vi "Plot_Many_Channels.vi"() -> (5 "Plug in titles":string[](array[string]), 7 "Plug in values":string[](array[string]))   [LabVIEW 2021]
uses:
  07834b75-344c-4d4c-a66e-07bf327eec95.vi
  Globals/Meas_global.vi
  <vilib>/Analysis/NI_AALBase.lvlib
panel:
  in  "Display:":enum16{"Show All", "My Choice", "Hide All"}(ring)
  in  "Plot:":enum16{"Eng. Units", "Voltages"}(ring)
  out "XY Graph":cluster{"Time (s)":dbl[], "Voltage":dbl[]}[](graph)
  # "Channel"
  # "Value"
  # "Voltage"
  # "StdDev(V)"
  # "Name"
  # "Symbol"
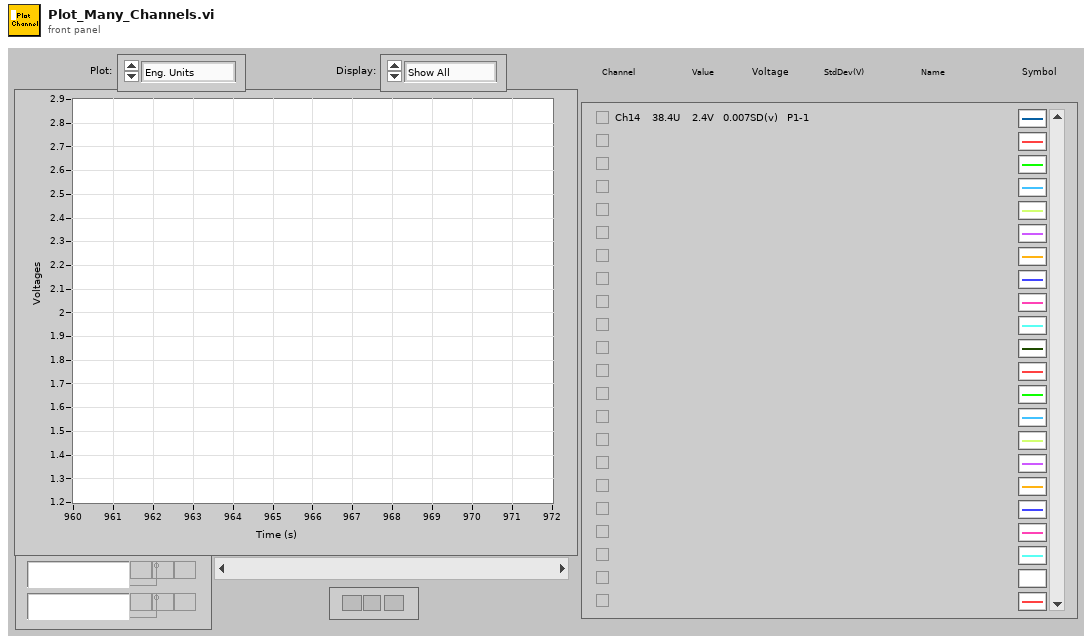
[diagram p1: front panel]
types:
  T1 = typedef "Analysis_info_cluster.ctl" = cluster{"Colour":u32, "Inst type":T2, "Inst name":string, "Symbol":string, "Code name":string, "Extra Info":string, "Inst Array":T3, "Extra Titles":string[], "Extra Values":string[], "U":dbl, "u^2":dbl, "u^3":dbl, "u^4":dbl, "Skew_u":dbl, "Kurt_u":dbl, "Sd Error in Mean":dbl, "% u'/U":dbl, "X":dbl, "Y":dbl, "Z":dbl, "Timescale integral Estimate":dbl, "Sd Error in Variance":dbl, "Calib File":path, "Calib Constants":dbl[], "Output Position":bool, "Stats":enum16{"None", "Basic", "Full"}, "Av Sampling Rate":dbl, "Av No of Samples":dbl, "Total Meas Time (s)":dbl, "ADAM Ch Name":string, "Max value":dbl, "Min value":dbl, "Req Sample Rate Hz":dbl, "Sync Delay Time (s)":dbl, "Ch No":i16, "Device":string, "Use Latest Calib":bool, "Port":string, "Metadata Ch Names":string[], "Metadata Ch Values":string[], "Label":string}
  T2 = typedef "Inst_type.ctl" = enum16{"Raw voltage", "Raw with zero offsetting", "Propeller anemometer", "Pressure Transducer", "Pitot-static tube", "Hot wire", "Cross wire 1", "Cross wire 2", "Generic Linear", "Generic Polynomial", "Generic BackPoly", "Fast FID", "Thermocouple", "Cold wire", "Pulsed Wire", "LDA Vel", "LDA Tran time", "LDA Arr time", "Microphone"}
  T3 = typedef "Instrument_Array.ctl" = enum16{"PWA", "LDA", "Analogue"}
  T4 = typedef "Time_Trace_Cluster.ctl" = cluster{"Weighting":dbl[], "Voltage":dbl[], "Eng Values":dbl[]}
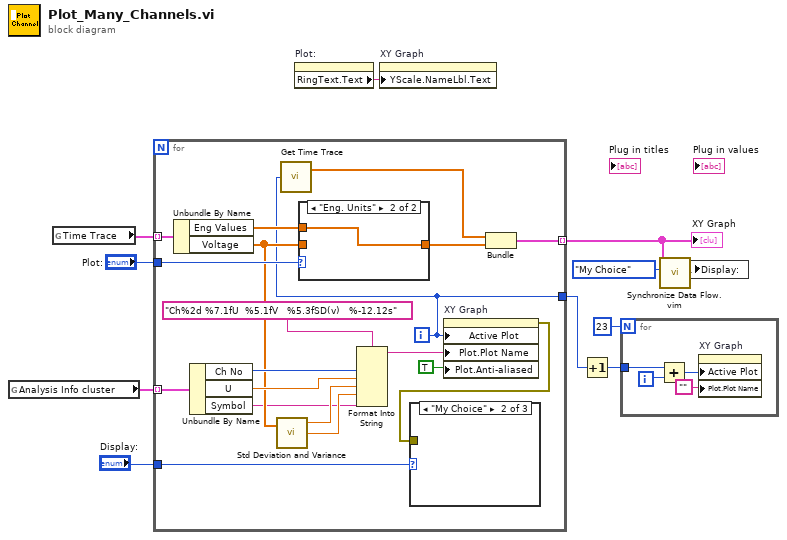
[diagram p0: block diagram]
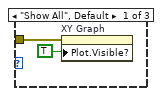
[diagram p2: hidden frame]
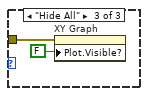
[diagram p3: hidden frame]
diagram:
  n1 = global read "Meas_global.vi" "Analysis Info cluster"() -> (w11:T1[])
  n2 = global read "Meas_global.vi" "Time Trace"() -> (w8:T4[])
  n3 = for {
    tunnel: [w30] -> w5 mode=indexing
    tunnel: w11 -> [w29] mode=indexing
    tunnel: "Plot:" -> [w28]
    tunnel: "Display:" -> [w15]
    tunnel: w8 -> [w14] mode=indexing
    tunnel: [w13] -> w3
    i -> [w13]
    n4 = Unbundle By Name(w14) -> ("Eng Values"=w21:dbl[], "Voltage"=w20:dbl[])
    n5 = Unbundle By Name(w29) -> ("Ch No"=w26:i16, "U"=w25:dbl, "Symbol"=w17:string)
    n6 = call <vilib>:"Std Deviation and Variance.vi"("X"=w20) -> ("mean"=w19:dbl, "standard deviation"=w18:dbl)  [unwired: 1 in, 1 out]
    n7 = call "Get Time Trace.vi"("Channel Index"=w13) -> ("Time (s)"=w12:dbl[])  [unwired: 1 out]
    n8 = case shown="\"Eng. Units\"" w28 {
      tunnel: [w35 w36] -> w22
      tunnel: w20 -> [w35 _]
      tunnel: w21 -> [_ w36]
      frame "Voltages" {
      }
      frame "Eng. Units" {
      }
    }
    n9 = Format Into String(format string="Ch%2d %7.1fU  %5.1fV   %5.3fSD(v)   %-12.12s", w26, w25, w19, w18, w17) -> (resulting string=w24:string)  [unwired: 2 in, 1 out]
    n10 = property on="XY Graph" class="XYGraph (strict)"("Active Plot"=w13, "Plot.Plot Name"=w24, "Plot.Anti-aliased"=TRUE) -> (error out=w16:errorcluster)  [unwired: 2 in, 1 out]
    n11 = case shown="\"My Choice\"" w15 {
      tunnel: w16 -> [w32 _ w34]
      frame "Show All", Default {
        n12 = property on="XY Graph" class="XYGraph (strict)"(error in=w32, "Plot.Visible?"=TRUE ("Plot.Visible")) -> ()  [unwired: 1 in, 2 out]
      }
      frame "My Choice" {
      }
      frame "Hide All" {
        n13 = property on="XY Graph" class="XYGraph (strict)"(error in=w34, "Plot.Visible?"=FALSE ("Plot.Visible")) -> ()  [unwired: 1 in, 2 out]
      }
    }
    n14 = Bundle("Time (s)"=w12, "Eng Values"=w22) -> (w30:cluster{"Time (s)":dbl[], "Eng Values":dbl[]})  [unwired: 1 in]
  }
  "XY Graph" <- w5
  n15 = property on="Plot:" class="Enum (strict)"() -> ("RingText.Text"=w1:string)  [unwired: 2 in, 2 out]
  n16 = property on="XY Graph" class="XYGraph (strict)"("YScale.NameLbl.Text"=w1) -> ()  [unwired: 2 in, 2 out]
  n17 = Increment(x=w3) -> (x+1=w2:i32)
  n18 = for {
    N: 23 -> [_]
    tunnel: w2 -> [w37]
    i -> [w38]
    n19 = Add(x=w37, y=w38) -> (x+y=w39:i32)
    n20 = property on="XY Graph" class="XYGraph (strict)"("Active Plot"=w39, "Plot.Plot Name"="") -> ()  [unwired: 2 in, 2 out]
  }
  n21 = call "Synchronize Data Flow.vim"("input 2"=enum16{"Show All", "My Choice", "Hide All"}."My Choice" ("show"), "input 1"=w5) -> ("output 2"=w6:enum16{"Show All", "My Choice", "Hide All"})  [unwired: 2 in, 3 out]
  n22 = local write "Display:"(w6) -> ()
